vi "TestStartSubRoutine.vi"() -> ()   [LabVIEW 2017]
uses:
  AutoSubsystem/AutoInput.ctl
  AutoSubsystem/AutoSubroutine.lvclass
panel:
  out "Local Start 3":timestamp
  out "Local Start 2":timestamp
  out "current time":timestamp
  out "Local Start":timestamp
  in  "GeneralAutoInput":T1
  out "Okay before both":bool
  out "Not okay after end by":bool
  out "Not okay after start by":bool
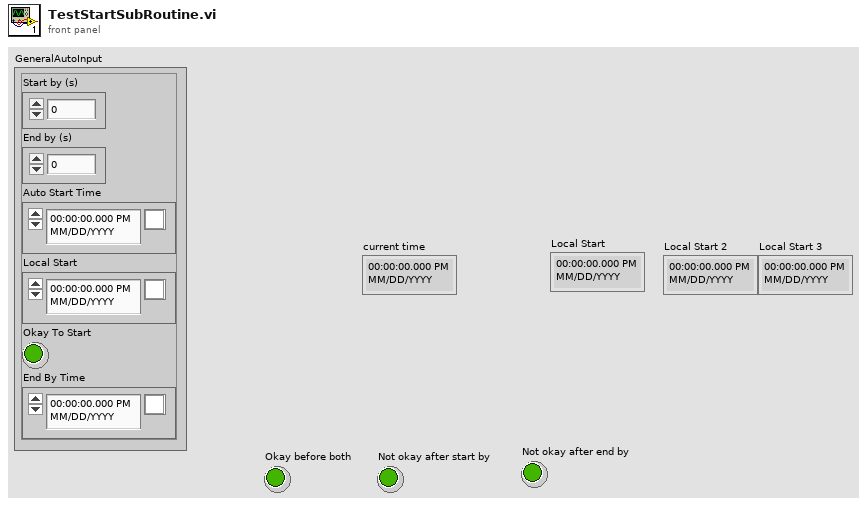
[diagram p1: front panel]
types:
  T1 = typedef "AutoSubroutine.lvclass/AutoInput.ctl" = cluster{"Start by (s)":dbl, "End by (s)":dbl, "Auto Start Time":timestamp, "Local Start":timestamp, "Okay To Start":bool, "End By Time":timestamp}
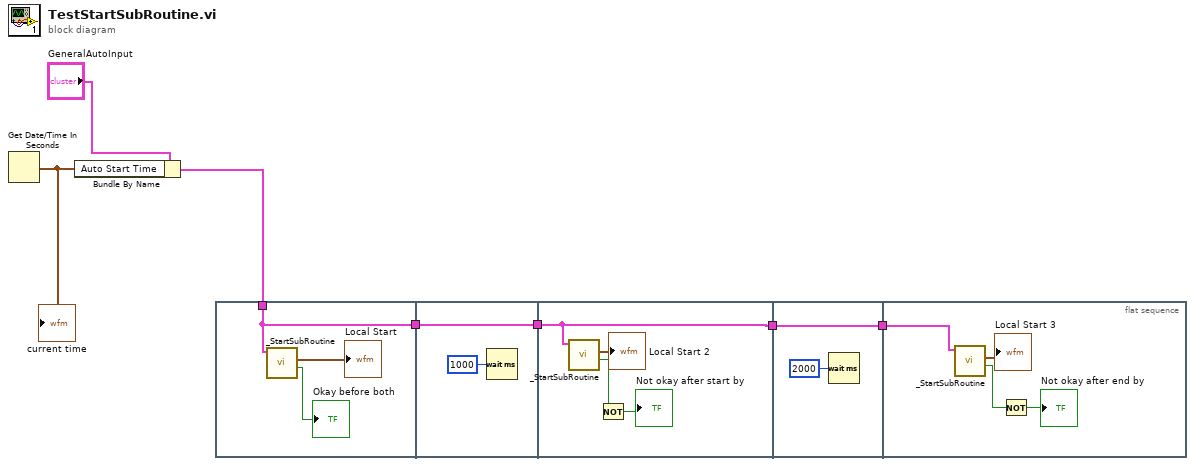
[diagram p0: block diagram]
diagram:
  n1 = Get Date/Time In Seconds() -> (seconds since 1Jan1904=w6:timestamp)
  "current time" <- w6
  n2 = Bundle By Name(cluster="GeneralAutoInput", "Auto Start Time"=w6) -> (w5:T1)
  n3 = flat-sequence {
    tunnel: w5 -> [w9]
    tunnel: [w9] -> w3
    tunnel: [w11] -> w4
    tunnel: w3 -> [w11]
    tunnel: w4 -> [w16]
    tunnel: [w16] -> w2
    tunnel: w2 -> [w18]
    tunnel: [w18] -> w1
    tunnel: w1 -> [w22]
    frame #0 {
      n4 = call "_StartSubRoutine.vi"("GeneralAutoInput"=w9) -> ("Okay to start?"=→"Okay before both":bool, "Local Start"=→"Local Start":timestamp)  [unwired: 7 in, 2 out]
    }
    frame #1 {
      n5 = Wait (ms)(milliseconds to wait=u32 1000) -> ()  [unwired: 1 out]
    }
    frame #2 {
      n6 = call "_StartSubRoutine.vi"("GeneralAutoInput"=w16) -> ("Okay to start?"=w14:bool, "Local Start"=→"Local Start 2":timestamp)  [unwired: 7 in, 2 out]
      n7 = Not(x=w14) -> (.not. x?=→"Not okay after start by":bool)
    }
    frame #3 {
      n8 = Wait (ms)(milliseconds to wait=u32 2000) -> ()  [unwired: 1 out]
    }
    frame #4 {
      n9 = call "_StartSubRoutine.vi"("GeneralAutoInput"=w22) -> ("Okay to start?"=w20:bool, "Local Start"=→"Local Start 3":timestamp)  [unwired: 7 in, 2 out]
      n10 = Not(x=w20) -> (.not. x?=→"Not okay after end by":bool)
    }
  }
